vi "initQueueAndEvent.vi"(8 "error in (no error)":errorcluster) -> (0 "error out":errorcluster, 1 "EventOut":T1, 3 "QueueOut":refnum<queue>)   [LabVIEW 2014]
doc: "- Tao User Event cho WhileLoop cua Modbus và mainloop event.\n- Tao queue Controller"
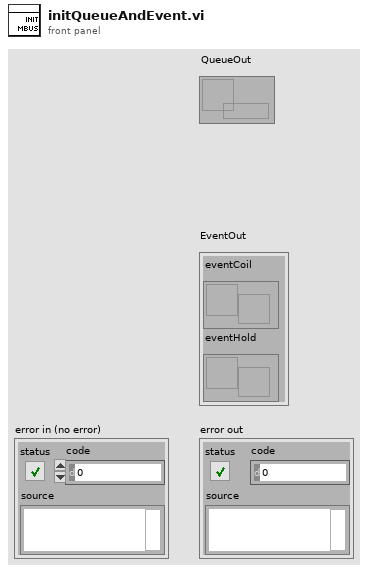
[diagram p1: front panel]
types:
  T1 = cluster{"eventCoil":refnum<user-event>, "eventHold":refnum<user-event>}
  T2 = cluster{"StartAddress":u16, "DataHold":u16[], "datacoil":bool, "AddressModbus":u16, "stateCMD":enum16{"WriteCoil", "WriteHold", "ChangeID", "Stop"}}
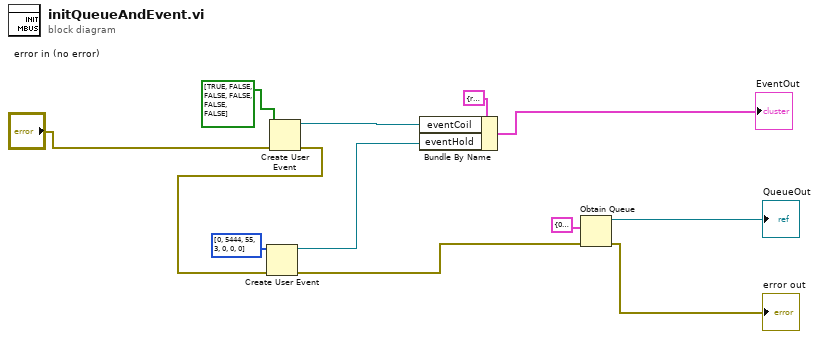
[diagram p0: block diagram]
diagram:
  n1 = Create User Event(user event datatype=bool[] [TRUE, FALSE, FALSE, FALSE, FALSE, FALSE] ("CoilChange"), error in="error in (no error)") -> (user event=w6:refnum<user-event>, error out=w9:errorcluster)
  n2 = Create User Event(user event datatype=u16[] [0, 5444, 55, 3, 0, 0, 0] ("HoldingChange"), error in=w9) -> (user event=w7:refnum<user-event>, error out=w11:errorcluster)
  n3 = Bundle By Name(cluster=T1 {"eventCoil"=refnum, "eventHold"=refnum} ("input cluster"), "eventCoil"=w6, "eventHold"=w7) -> (→"EventOut":T1)
  n4 = Obtain Queue(element data type=T2 {"StartAddress"=0, "DataHold"=[3, 544, 35200, 3], "datacoil"=FALSE, "AddressModbus"=0, "stateCMD"=enum."WriteCoil"}, error in (no error)=w11) -> (queue out=→"QueueOut":refnum<queue>, error out=→"error out":errorcluster)  [unwired: 3 in, 1 out]
